vi "FFT (single).vi"(8 "error in (no error)":errorcluster, 11 "XY-data":cluster{"X-array":dbl[], "Y-array":dbl[]} {"Y-array" format="%.2p"; "X-array" format="%.2p"}) -> (0 "error out":errorcluster, 1 "phase":cluster{"f0":dbl, "df":dbl, "phase":dbl[]} {"phase" format="%.2p"; "f0" format="%0.2p"; "df" format="%0.2p"}, 2 "magnitude":cluster{"f0":dbl, "df":dbl, "magnitude":dbl[]} {"magnitude" format="%.2p"; "f0" format="%0.2p"; "df" format="%0.2p"}, 3 "XY-data out":cluster{"X-array":dbl[], "Y-array":dbl[]} {"Y-array" format="%.2p"; "X-array" format="%.2p"})   [LabVIEW 2019, in "xy_utilities.lvlib"]
doc: "Computes the FFT spectrum of <B>XY-data</B>. This VI returns the FFT results as <B>magnitude</B> and <B>phase</B>. This VI is a wrapper for NI_MAPro.lvlib:FFT Spectrum (Mag-Phase).vi\n\nWire data to the data input to determine the polymorphic instance to use or manually select the instance."
uses:
  xy_utilities.lvlib
  Get X and Y.vi
  Get X and Y (single).vi
  Resample.vi
  Resample (single).vi
  Private/Get X Array dx.vi
  <vilib>/measure/maresamp.llb/Resample Waveforms (single shot).vi
  <vilib>/measure/maresamp.llb/Resample Pair of Arrays (single shot).vi
  <vilib>/measure/maspectr.llb/FFT Spectrum (Mag-Phase) for 1 Chan.vi
  <vilib>/measure/NI_MAPro.lvlib
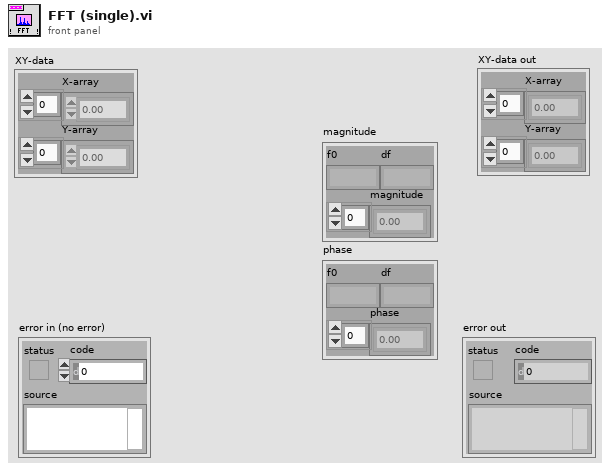
[diagram p1: front panel]
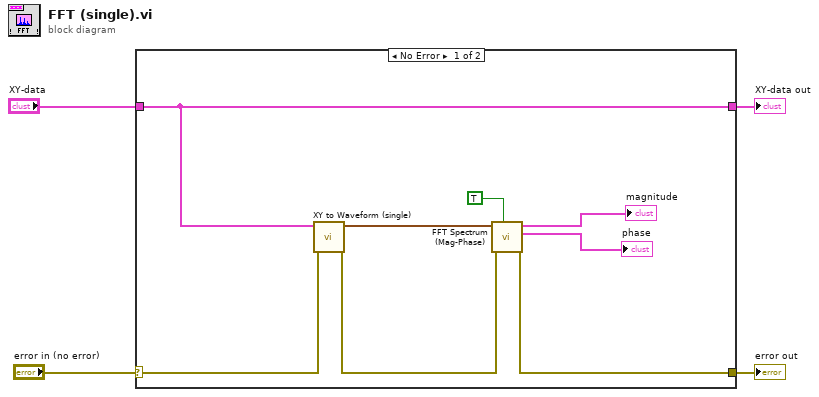
[diagram p0: block diagram]
diagram:
  n1 = case shown="No Error" "error in (no error)" {
    selector: "error in (no error)" -> [w6 w14]
    tunnel: [w10 w14] -> w3
    tunnel: "XY-data" -> [w8 w13]
    tunnel: [w8 w13] -> w1
    frame No Error {
      n2 = call "XY to Waveform (single).vi"("error in (no error)"=w6, "XY-data in"=w8) -> ("error out"=w5:errorcluster, "Waveform out"=w7:waveform(dbl))  [unwired: 7 in, 1 out]
      n3 = call-poly <vilib>:"FFT Spectrum (Mag-Phase).vi"("restart averaging (F)"=TRUE, "error in (no error)"=w5, "time signal"=w7) -> ("error out"=w10:errorcluster, "phase"=→"phase":cluster{"f0":dbl, "df":dbl, "phase":dbl[]}, "magnitude"=→"magnitude":cluster{"f0":dbl, "df":dbl, "magnitude":dbl[]})  [unwired: 4 in, 2 out]
    }
    frame Error {
    }
  }
  "error out" <- w3
  "XY-data out" <- w1
